vi "Untitled 3.vi"() -> ()   [LabVIEW 2017]
uses:
  <vilib>/Platform/TimedLoop/XDataNode/timing_clust.ctl
  <vilib>/Platform/TimedLoop/XDataNode/nitl_modes.ctl
  <vilib>/Platform/TimedLoop/XDataNode/wakeup.ctl
  <vilib>/myRIO/Common/Instrument Driver Framework/myRIO v1.0/UART/vis/myRIO v1.0 Close UART.vi
  Projects/Auto control/Global 1.vi
  Projects/Auto control/Outputs.vi
  Projects/Auto control/Inputs.vi
  <vilib>/myRIO/Common/Instrument Driver Framework/Utilities/vis/FPGA Ref Manager.vi
  <vilib>/myRIO/Common/Instrument Driver Framework/myRIO v1.0/myRIO v1.0 Reset FPGA.vi
  <vilib>/myRIO/Common/Instrument Driver Framework/myRIO v1.0/IRQ/vis/myRIO v1.0 IRQ Info FGV.vi
  <vilib>/myRIO/Common/Instrument Driver Framework/myRIO v1.0/IRQ/vis/myRIO v1.0 Timer IRQ Info FGV.vi
  <vilib>/myRIO/Common/Instrument Driver Framework/myRIO v1.0/IRQ/vis/myRIO v1.0 ISR Agent.vi
  <vilib>/platform/TimedLoop/XDataNode/XDataNode.xnode
  <vilib>/Platform/TimedLoop/XDataNode/XDNodeRunTimeDep.lvlib
  <vilib>/myRIO/Instrument Drivers/Utilities/Utilities.lvlib
panel:
  out "error out":errorcluster
  in  "Stop":bool
  out "Step":i16
  in  "Start":bool
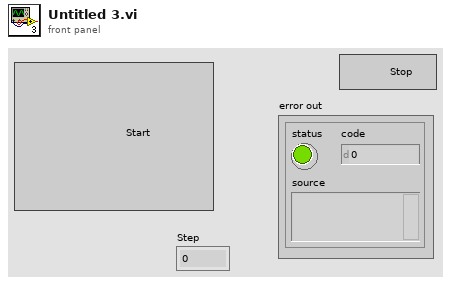
[diagram p1: front panel]
types:
  T1 = typedef "XDNodeRunTimeDep.lvlib/timing_clust.ctl" = cluster{"Expected End [f-1]":u64, "Actual End [f-1]":u64, "Finished Late? [f-1]":bool, "Expected End [i-1]":u64, "Actual End [i-1]":u64, "Finished Late? [i-1]":bool, "Expected Start [i]":u64, "Actual Start [i]":u64, "Expected Start [f]":u64, "Actual Start [f]":u64, "Source Name":string, "Structure Name":string, "Period":i64, "Deadline":i64, "Offset":i64, "Start":i64, "Priority":i32, "Timeout":i32, "Mode":T2, "Wakeup Reason":T3, "Error":errorcluster, "Source Type":string, "Secondary Source Type":string, "Global End Time":u64, "Global Start Time":u64, "Frame Duration":u64, "Iteration Duration":u64, "Assigned CPU":i32, "I/O Scan Engine Mode":u32}
  T2 = typedef "XDNodeRunTimeDep.lvlib/nitl_modes.ctl" = enum32{"No Change", "Process missed periods, maintain original phase", "Discard missed periods, maintain original phase", "Process missed periods, ignore original phase", "Discard missed periods, ignore original phase"}
  T3 = typedef "XDNodeRunTimeDep.lvlib/wakeup.ctl" = enum32{"Normal", "Aborted", "Asynchronous wakeup", "Timing source error", "Timed loop error", "Timeout"}
  T4 = typedef "I2C.lvlib/I2C Reference.ctl" = cluster{"myRIO Reference":T5, "I2C Channels Enum":T9, "I2C Configuration":T10}
  T5 = typedef "myRIO Generic Hardware Reference.ctl" = cluster{"myRIO Model":T6, "myRIO Hardware Reference":T7}
  T6 = typedef "Hardware Version Enum.ctl" = enum16{"Unknown", "myRIO-1900", "myRIO-1950", "roboRIO", "NI ELVIS RIO CM"}
  T7 = typedef "myRIO v1.0 Reference.ctl" = cluster{"Generic FPGA Reference":T8, "Allow multiple opens":bool}
  T8 = typedef "Generic FPGA Reference.ctl" = refnum<k20>
  T9 = typedef "I2C Channels Enum.ctl" = enum16{"Not Connected", "A/I2C", "B/I2C", "I2C/I2C"}
  T10 = typedef "I2C.lvlib/I2C Configuration.ctl" = cluster{"I2C Transfer Rate":T11}
  T11 = typedef "I2C.lvlib/I2C Transfer Rate.ctl" = enum16{"Standard mode (100 kbps)", "Fast mode (400 kbps)"}
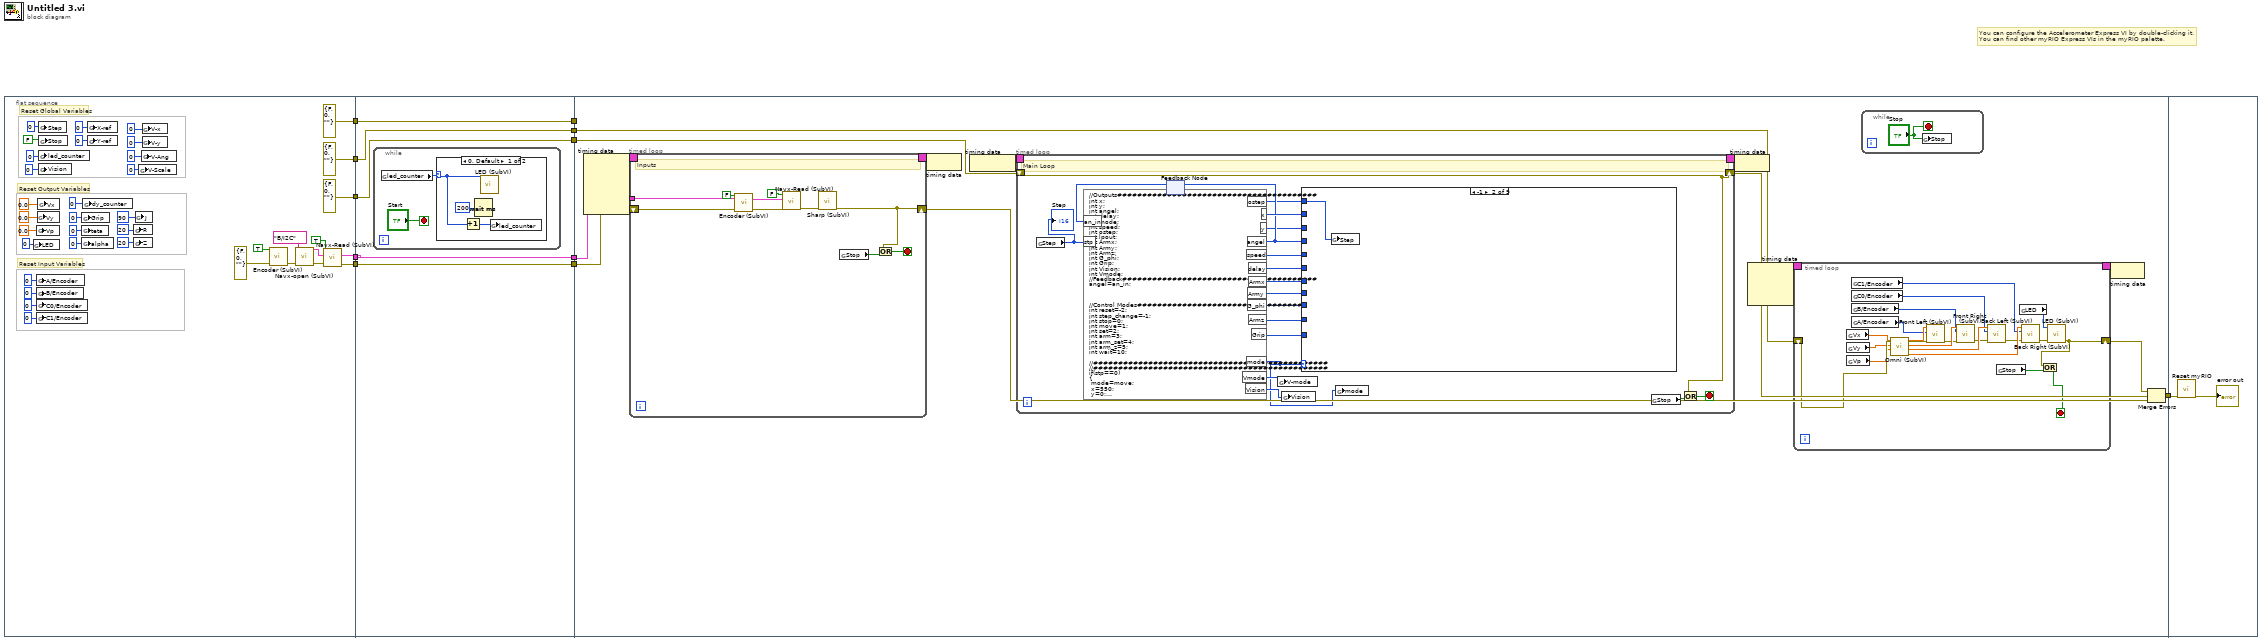
[diagram p0: block diagram]
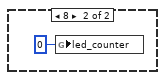
[diagram p2: hidden frame]
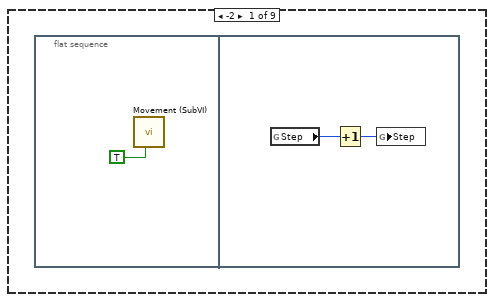
[diagram p3: hidden frame]
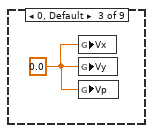
[diagram p4: hidden frame]
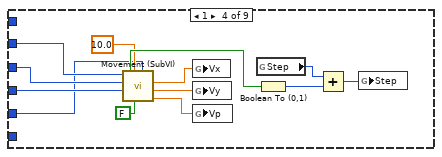
[diagram p5: hidden frame]
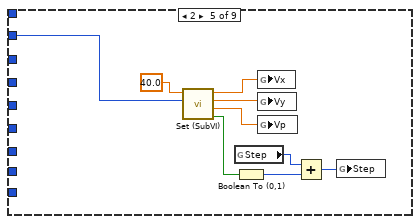
[diagram p6: hidden frame]
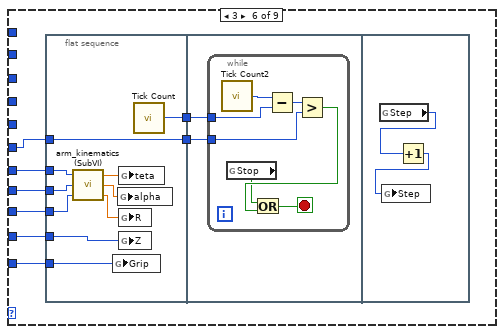
[diagram p7: hidden frame]
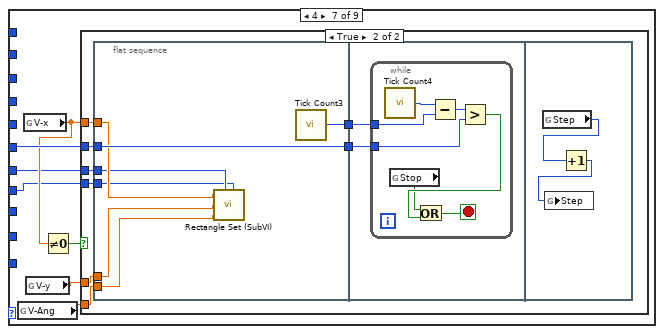
[diagram p8: hidden frame]
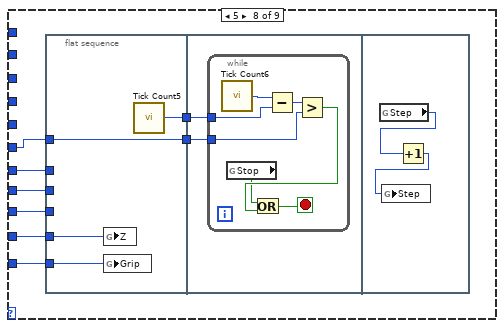
[diagram p10: hidden frame]
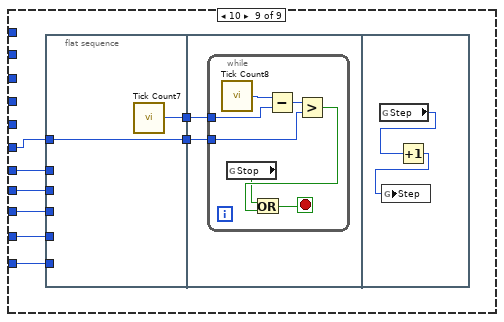
[diagram p11: hidden frame]
diagram:
  # "You can configure the Accelerometer Express VI by double-clicking it.\nYou can find other myRIO Express VIs in the myRIO palette."
  n1 = flat-sequence {
    tunnel: [w43] -> w11
    tunnel: [errorcluster {"status"=FALSE, "code"=0, "source"=""} ("error in (no error)")] -> w10
    tunnel: [errorcluster {"status"=FALSE, "code"=0, "source"=""} ("error in (no error)")] -> w9
    tunnel: [w41] -> w8
    tunnel: [errorcluster {"status"=FALSE, "code"=0, "source"=""} ("error in (no error)")] -> w7
    tunnel: w11 -> [w52]
    tunnel: [w52] -> w6
    tunnel: w10 -> [w51]
    tunnel: [w51] -> w5
    tunnel: w9 -> [w48]
    tunnel: w8 -> [w50]
    tunnel: [w50] -> w4
    tunnel: [w49] -> w3
    tunnel: w7 -> [w49]
    tunnel: [w48] -> w2
    tunnel: w6 -> [w72]
    tunnel: w5 -> [_]
    tunnel: w4 -> [w65]
    tunnel: w3 -> [w64]
    tunnel: [w63] -> w1
    tunnel: w2 -> [w59]
    tunnel: w1 -> [w267]
    frame #0 {
      # "Reset Global Variables"
      # "Reset Input Variables"
      # "Reset Output Variables"
      # "Initialize"
      n2 = global write "Outputs.vi" "LED"(i8 0 ("LED")) -> ()
      n3 = global write "Outputs.vi" "Vp"(0.0 ("Vp")) -> ()
      n4 = global write "Inputs.vi" "A/Encoder"(0 ("A/Encoder")) -> ()
      n5 = global write "Inputs.vi" "B/Encoder"(0 ("B/Encoder")) -> ()
      n6 = global write "Inputs.vi" "C0/Encoder"(0 ("C0/Encoder")) -> ()
      n7 = global write "Inputs.vi" "C1/Encoder"(0 ("C1/Encoder")) -> ()
      n8 = global write "Outputs.vi" "Vy"(0.0 ("Vy")) -> ()
      n9 = global write "Outputs.vi" "Vx"(0.0 ("Vx")) -> ()
      n10 = global write "Global 1.vi" "Step"(i16 0 ("Step")) -> ()
      n11 = global write "Global 1.vi" "led_counter"(i8 0 ("Step")) -> ()
      n12 = global write "Global 1.vi" "Vision"(i8 0 ("Step")) -> ()
      n13 = global write "Global 1.vi" "Stop"(FALSE ("Stop")) -> ()
      n14 = global write "Outputs.vi" "Grip"(i16 0 ("Grip")) -> ()
      n15 = global write "Outputs.vi" "teta"(i16 0 ("teta")) -> ()
      n16 = global write "Outputs.vi" "alpha"(i16 0 ("alpha")) -> ()
      n17 = global write "Outputs.vi" "dy_counter"(i8 0 ("LED")) -> ()
      n18 = global write "Global 1.vi" "X-ref"(i64 0 ("X-ref")) -> ()
      n19 = global write "Global 1.vi" "Y-ref"(i64 0 ("Y-ref")) -> ()
      n20 = global write "Outputs.vi" "R"(i16 20 ("R")) -> ()
      n21 = global write "Outputs.vi" "Z"(i16 20 ("Z")) -> ()
      n22 = global write "Outputs.vi" "J"(i16 90 ("J")) -> ()
      n23 = global write "Global 1.vi" "V-Scale"(i64 0 ("Y-ref")) -> ()
      n24 = global write "Global 1.vi" "V-Ang"(i64 0 ("X-ref")) -> ()
      n25 = global write "Global 1.vi" "V-x"(i64 0 ("X-ref")) -> ()
      n26 = global write "Global 1.vi" "V-y"(i64 0 ("Y-ref")) -> ()
      n27 = call "Encoder (SubVI).vi"("error in (no error)"=errorcluster {"status"=FALSE, "code"=0, "source"=""}, "Reset?"=TRUE ("Reset Counter")) -> ("error out"=w25:errorcluster)  [unwired: 9 in]
      n28 = call "Navx-open (SubVI).vi"("error in (no error)"=w25, "Channel Name"=tag "B/I2C") -> ("error out"=w45:errorcluster, "I2C Ref Out"=w41:T4)  [unwired: 8 in]
      n29 = call "Navx-Read (SubVI).vi"("error in (no error)"=w45, "I2C Ref Out"=w41, "Reset"=TRUE) -> ("error out"=w43:errorcluster)  [unwired: 7 in, 1 out]
    }
    frame #1 {
      n30 = while {
        stop <- "Start" stop-if-true
        n31 = global read "Global 1.vi" "led_counter"() -> (w53:i8)
        n32 = case shown="0, Default" w53 {
          selector: w53 -> [w55 _]
          frame 0, Default {
            n33 = Increment(x=w55) -> (x+1=w57:i8)
            n34 = Wait (ms)(milliseconds to wait=u32 200) -> ()  [unwired: 1 out]
            n35 = call "LED (SubVI).vi"("LED"=w55) -> ()  [unwired: 10 in, 1 out]
            n36 = global write "Global 1.vi" "led_counter"(w57) -> ()
          }
          frame 8 {
            n37 = global write "Global 1.vi" "led_counter"(i8 0 ("led_counter")) -> ()
          }
        }
      }
    }
    frame #2 {
      n38 = node-c288() -> (w67:T1)  [unwired: 5 in]
      n39 = timed-loop {
        shift-right: [w77] -> w62
        shift-left: w72 -> [w81]
        timing: w67 -> [_]
        timing-out: [_] -> w66
        tunnel: w65 -> [w79]
        stop <- w80 stop-if-true
        # "Inputs"
        n40 = call "Encoder (SubVI).vi"("error in (no error)"=w81, "Reset?"=FALSE ("Boolean")) -> ("error out"=w75:errorcluster)  [unwired: 9 in]
        n41 = call "Navx-Read (SubVI).vi"("error in (no error)"=w75, "I2C Ref Out"=w79, "Reset"=FALSE) -> ("error out"=w74:errorcluster)  [unwired: 7 in, 1 out]
        n42 = call "Sharp (SubVI).vi"("error in (no error)"=w74) -> ("error out"=w77:errorcluster)  [unwired: 10 in]
        n43 = global read "Global 1.vi" "Stop"() -> (w78:bool)
        n44 = Or(x=w77, y=w78) -> (x .or. y?=w80:bool)
      }
      n45 = node-c288(w66) -> ()
      n46 = node-c288() -> (w69:T1)
      n47 = timed-loop {
        shift-right: [w103] -> w61
        shift-left: w59 -> [w103]
        timing: w69 -> [_]
        timing-out: [_] -> w68
        stop <- w104 stop-if-true
        # "Main Loop"
        n48 = global read "Global 1.vi" "Step"() -> (w96:i16)
        "Step" <- w96
        n49 = feedback #1() -> (w100:i32)  [unwired: 1 in]
        n50 = formula code="//Outputs########################################\nint x;\nint y;\nint angel;\nint delay;\nint mode;\nint speed;\nint ostep;\nint lpout;\nint Armx;\nint Army;\nint Armz;\nint G_phi;\nint Grip;\nint Vision;\nint Vmode;\n//Feedback#######################################\nangel=an_in;\n\n\n\n//Control Modes##################################\nint reset=-2;\nint step_change=-1; \nint stop=0;\nint move=1;\nint set=2;\nint arm=3;\nint arm_set=4;\nint arm_z=5;\nint wait=10;\n\n//###############################################\n//###############################################\nif(stp==0)\n{\n\tmode=move;\n\tx=550;\n\ty=0;\n\tangel=0;\n\tspeed=100;\n}\nif(stp==1)\n{\n\tmode=move;\n\tx=0;\n\ty=-1400;\n\tangel=0;\n\tspeed=100;\n}\nif(stp==2)\n{\n\tmode=move;\n\tx=1400;\n\ty=0;\n\tangel=0;\n\tspeed=100;\n}\nif(stp==3)\n{\n\tmode=move;\n\tx=0;\n\ty=1400;\n\tangel=0;\n\tspeed=100;\n}\nif(stp==4)\n{\n\tmode=move;\n\tx=2000;\n\ty=0;\n\tangel=0;\n\tspeed=100;\n}\nif(stp==5)\n{\n\tmode=move;\n\tx=0;\n\ty=-1000;\n\tangel=0;\n\tspeed=100;\n}\nif(stp==6)\n{\n\tmode=move;\n\tx=2000;\n\ty=0;\n\tangel=0;\n\tspeed=100;\n}\nif(stp==7)\n{\n\tmode=move;\n\tx=0;\n\ty=0;\n\tangel=-90;\n\tspeed=100;\n}\nif(stp==8)\n{\n\tmode=move;\n\tx=4000;\n\ty=0;\n\tangel=0;\n\tspeed=100;\n}\n\n\nif(stp==9)\n{\n\tmode=stop;\n}"("stp"=w96, "an_in"=w100) -> ("x"=w102:i32, "y"=w97:i32, "mode"=w86:i32, "angel"=w99:i32, "delay"=w101:i32, "speed"=w98:i32, "ostep"=w94:i32, "Armx"=w92:i32, "Army"=w91:i32, "Armz"=w90:i32, "G_phi"=w93:i32, "Grip"=w89:i32, "Vision"=w88:i32, "Vmode"=w87:i32)
        n51 = feedback-in #1(w99) -> ()
        n52 = global write "Global 1.vi" "V-mode"(w87) -> ()
        n53 = global write "Global 1.vi" "Vision"(w88) -> ()
        n54 = case shown="-1" w86 {
          tunnel: w102 -> [_ _ _ w116 w131 _ _ _ _]
          tunnel: w97 -> [_ _ _ w115 _ _ _ _ _]
          tunnel: w99 -> [_ _ _ w114 _ _ _ _ _]
          tunnel: w101 -> [_ _ _ _ _ w138 w167 w200 w223]
          tunnel: w98 -> [_ _ _ w113 _ _ _ _ _]
          tunnel: w94 -> [_ w108 _ _ _ _ _ _ _]
          tunnel: w93 -> [_ _ _ _ _ w134 _ w196 w219]
          tunnel: w92 -> [_ _ _ _ _ w136 w162 w198 w221]
          tunnel: w91 -> [_ _ _ _ _ w135 w161 w197 w220]
          tunnel: w90 -> [_ _ _ _ _ w133 _ w195 w218]
          tunnel: w89 -> [_ _ _ _ _ w132 _ w194 w217]
          frame -2 {
            n55 = flat-sequence {
              frame #0 {
                n56 = call "Movement (SubVI).vi"("Reset"=TRUE) -> ()  [unwired: 6 in, 4 out]
              }
              frame #1 {
                n57 = global read "Global 1.vi" "Step"() -> (w107:i16)
                n58 = Increment(x=w107) -> (x+1=w106:i16)
                n59 = global write "Global 1.vi" "Step"(w106) -> ()
              }
            }
          }
          frame -1 {
            n60 = global write "Global 1.vi" "Step"(w108) -> ()
          }
          frame 0, Default {
            w109 = 0.0 ("Vy")
            n61 = global write "Outputs.vi" "Vx"(w109) -> ()
            n62 = global write "Outputs.vi" "Vy"(w109) -> ()
            n63 = global write "Outputs.vi" "Vp"(w109) -> ()
          }
          frame 1 {
            n64 = call "Movement (SubVI).vi"("Speed"=w113, "Reset"=FALSE, "Acc"=10.0, "Goal P"=w114, "Goal Y"=w115, "Goal X"=w116) -> ("Vp"=w118:dbl, "Vy"=w119:dbl, "Vx"=w120:dbl, "Reach?"=w121:bool)  [unwired: 1 in]
            n65 = global write "Outputs.vi" "Vx"(w120) -> ()
            n66 = global write "Outputs.vi" "Vy"(w119) -> ()
            n67 = global write "Outputs.vi" "Vp"(w118) -> ()
            n68 = global read "Global 1.vi" "Step"() -> (w110:i16)
            n69 = Boolean To (0,1)(Boolean=w121) -> (0, 1=w122:i16)
            n70 = Add(x=w110, y=w122) -> (x+y=w111:i16)
            n71 = global write "Global 1.vi" "Step"(w111) -> ()
          }
          frame 2 {
            n72 = call "Set (SubVI).vi"("Mode"=w131, "speed"=40.0) -> ("Reach?"=w123:bool, "Vp"=w127:dbl, "Vy"=w128:dbl, "Vx"=w129:dbl)  [unwired: 4 in]
            n73 = global read "Global 1.vi" "Step"() -> (w124:i16)
            n74 = Boolean To (0,1)(Boolean=w123) -> (0, 1=w126:i16)
            n75 = global write "Outputs.vi" "Vx"(w129) -> ()
            n76 = global write "Outputs.vi" "Vy"(w128) -> ()
            n77 = global write "Outputs.vi" "Vp"(w127) -> ()
            n78 = Add(x=w124, y=w126) -> (x+y=w125:i16)
            n79 = global write "Global 1.vi" "Step"(w125) -> ()
          }
          frame 3 {
            n80 = flat-sequence {
              tunnel: [w149] -> w139
              tunnel: w138 -> [w145]
              tunnel: [w145] -> w137
              tunnel: w136 -> [w144]
              tunnel: w135 -> [w143]
              tunnel: w134 -> [w142]
              tunnel: w133 -> [w141]
              tunnel: w132 -> [w140]
              tunnel: w139 -> [w151]
              tunnel: w137 -> [w150]
              frame #0 {
                n81 = call "arm_kinematics (SubVI).vi"("alpha"=w142, "y"=w143, "x"=w144) -> ("R"=w146:dbl, "alpha"=w147:dbl, "teta"=w148:dbl)
                n82 = global write "Outputs.vi" "Grip"(w140) -> ()
                n83 = global write "Outputs.vi" "alpha"(w147) -> ()
                n84 = global write "Outputs.vi" "teta"(w148) -> ()
                n85 = global write "Outputs.vi" "R"(w146) -> ()
                n86 = global write "Outputs.vi" "Z"(w141) -> ()
                n87 = call "Tick Count"() -> ("Tick Count(mSec)"=w149:u32)
              }
              frame #1 {
                n88 = while {
                  tunnel: w151 -> [w157]
                  tunnel: w150 -> [w152]
                  stop <- w154 stop-if-true
                  n89 = call "Tick Count2"() -> ("Tick Count(mSec)"=w158:u32)
                  n90 = global read "Global 1.vi" "Stop"() -> (w153:bool)
                  n91 = Subtract(x=w158, y=w157) -> (x-y=w156:u32)
                  n92 = Greater?(x=w156, y=w152) -> (0:w155:bool)
                  n93 = Or(x=w153, y=w155) -> (x .or. y?=w154:bool)
                }
              }
              frame #2 {
                n94 = global read "Global 1.vi" "Step"() -> (w159:i16)
                n95 = Increment(x=w159) -> (x+1=w160:i16)
                n96 = global write "Global 1.vi" "Step"(w160) -> ()
              }
            }
          }
          frame 4 {
            n97 = global read "Global 1.vi" "V-Ang"() -> (w163:sgl)
            n98 = global read "Global 1.vi" "V-x"() -> (w164:sgl)
            n99 = global read "Global 1.vi" "V-y"() -> (w166:sgl)
            n100 = Not Equal To 0?(x=w164) -> (x != 0?=w165:bool)
            n101 = case shown="True" w165 {
              tunnel: w167 -> [_ w173]
              tunnel: w166 -> [_ w172]
              tunnel: w164 -> [_ w171]
              tunnel: w163 -> [_ w170]
              tunnel: w162 -> [_ w169]
              tunnel: w161 -> [_ w168]
              frame False {
              }
              frame True {
                n102 = flat-sequence {
                  tunnel: [w182] -> w175
                  tunnel: w173 -> [w181]
                  tunnel: [w181] -> w174
                  tunnel: w172 -> [w179]
                  tunnel: w171 -> [w180]
                  tunnel: w170 -> [w178]
                  tunnel: w169 -> [w177]
                  tunnel: w168 -> [w176]
                  tunnel: w175 -> [w184]
                  tunnel: w174 -> [w183]
                  frame #0 {
                    n103 = call "Rectangle Set (SubVI).vi"("x"=w180, "x in"=w177, "y"=w179, "alpha"=w178, "y in"=w176) -> ()  [unwired: 6 in]
                    n104 = call "Tick Count3"() -> ("Tick Count(mSec)"=w182:u32)
                  }
                  frame #1 {
                    n105 = while {
                      tunnel: w184 -> [w190]
                      tunnel: w183 -> [w185]
                      stop <- w187 stop-if-true
                      n106 = call "Tick Count4"() -> ("Tick Count(mSec)"=w191:u32)
                      n107 = global read "Global 1.vi" "Stop"() -> (w186:bool)
                      n108 = Subtract(x=w191, y=w190) -> (x-y=w189:u32)
                      n109 = Greater?(x=w189, y=w185) -> (0:w188:bool)
                      n110 = Or(x=w186, y=w188) -> (x .or. y?=w187:bool)
                    }
                  }
                  frame #2 {
                    n111 = global read "Global 1.vi" "Step"() -> (w192:i16)
                    n112 = Increment(x=w192) -> (x+1=w193:i16)
                    n113 = global write "Global 1.vi" "Step"(w193) -> ()
                  }
                }
              }
            }
          }
          frame 5 {
            n114 = flat-sequence {
              tunnel: [w205] -> w201
              tunnel: w200 -> [w204]
              tunnel: [w204] -> w199
              tunnel: w198 -> [_]
              tunnel: w197 -> [_]
              tunnel: w196 -> [_]
              tunnel: w195 -> [w203]
              tunnel: w194 -> [w202]
              tunnel: w201 -> [w207]
              tunnel: w199 -> [w206]
              frame #0 {
                n115 = global write "Outputs.vi" "Z"(w203) -> ()
                n116 = global write "Outputs.vi" "Grip"(w202) -> ()
                n117 = call "Tick Count5"() -> ("Tick Count(mSec)"=w205:u32)
              }
              frame #1 {
                n118 = while {
                  tunnel: w207 -> [w213]
                  tunnel: w206 -> [w208]
                  stop <- w210 stop-if-true
                  n119 = call "Tick Count6"() -> ("Tick Count(mSec)"=w214:u32)
                  n120 = global read "Global 1.vi" "Stop"() -> (w209:bool)
                  n121 = Subtract(x=w214, y=w213) -> (x-y=w212:u32)
                  n122 = Greater?(x=w212, y=w208) -> (0:w211:bool)
                  n123 = Or(x=w209, y=w211) -> (x .or. y?=w210:bool)
                }
              }
              frame #2 {
                n124 = global read "Global 1.vi" "Step"() -> (w215:i16)
                n125 = Increment(x=w215) -> (x+1=w216:i16)
                n126 = global write "Global 1.vi" "Step"(w216) -> ()
              }
            }
          }
          frame 10 {
            n127 = flat-sequence {
              tunnel: [w226] -> w224
              tunnel: w223 -> [w225]
              tunnel: [w225] -> w222
              tunnel: w221 -> [_]
              tunnel: w220 -> [_]
              tunnel: w219 -> [_]
              tunnel: w218 -> [_]
              tunnel: w217 -> [_]
              tunnel: w224 -> [w228]
              tunnel: w222 -> [w227]
              frame #0 {
                n128 = call "Tick Count7"() -> ("Tick Count(mSec)"=w226:u32)
              }
              frame #1 {
                n129 = while {
                  tunnel: w228 -> [w234]
                  tunnel: w227 -> [w229]
                  stop <- w231 stop-if-true
                  n130 = call "Tick Count8"() -> ("Tick Count(mSec)"=w235:u32)
                  n131 = global read "Global 1.vi" "Stop"() -> (w230:bool)
                  n132 = Subtract(x=w235, y=w234) -> (x-y=w233:u32)
                  n133 = Greater?(x=w233, y=w229) -> (0:w232:bool)
                  n134 = Or(x=w230, y=w232) -> (x .or. y?=w231:bool)
                }
              }
              frame #2 {
                n135 = global read "Global 1.vi" "Step"() -> (w236:i16)
                n136 = Increment(x=w236) -> (x+1=w237:i16)
                n137 = global write "Global 1.vi" "Step"(w237) -> ()
              }
            }
          }
        }
        n138 = global write "Global 1.vi" "mode"(w86) -> ()
        n139 = global read "Global 1.vi" "Stop"() -> (w95:bool)
        n140 = Or(x=w103, y=w95) -> (x .or. y?=w104:bool)
      }
      n141 = node-c288(w68) -> ()
      n142 = node-c288() -> (w71:T1)  [unwired: 3 in]
      n143 = timed-loop {
        timing: w71 -> [_]
        timing-out: [_] -> w70
        shift-right: [w259] -> w60
        shift-left: w64 -> [w260]
        stop <- w261 stop-if-true
        n144 = global read "Outputs.vi" "Vx"() -> (w255:dbl)
        n145 = global read "Outputs.vi" "Vy"() -> (w257:dbl)
        n146 = global read "Outputs.vi" "Vp"() -> (w256:dbl)
        n147 = global read "Inputs.vi" "C1/Encoder"() -> (w248:i32)
        n148 = global read "Inputs.vi" "C0/Encoder"() -> (w247:i32)
        n149 = global read "Inputs.vi" "B/Encoder"() -> (w246:i32)
        n150 = global read "Inputs.vi" "A/Encoder"() -> (w245:i32)
        n151 = call "Omni (SubVI).vi"("Vp"=w256, "Vy"=w257, "Vx"=w255) -> ("Back_Right"=w253:dbl, "Back_Left"=w258:dbl, "Front_Right"=w254:dbl, "Front_Left"=w251:dbl)  [unwired: 4 in]
        n152 = call "Front Left (SubVI).vi"("setpoint"=w251, "Counter Value"=w245, "error in"=w260) -> ("error out"=w252:errorcluster)  [unwired: 6 in, 1 out]
        n153 = call "Front Right (SubVI).vi"("error in"=w252, "Counter Value"=w246, "setpoint"=w254) -> ("error out"=w250:errorcluster)  [unwired: 7 in, 1 out]
        n154 = call "Back Left (SubVI).vi"("error in"=w250, "Counter Value"=w247, "setpoint"=w258) -> ("error out"=w249:errorcluster)  [unwired: 7 in, 1 out]
        n155 = global read "Global 1.vi" "Stop"() -> (w244:bool)
        n156 = global read "Outputs.vi" "LED"() -> (w242:i8)
        n157 = call "Back Right (SubVI).vi"("error in"=w249, "Counter Value"=w248, "setpoint"=w253) -> ("error out"=w243:errorcluster)  [unwired: 7 in, 1 out]
        n158 = call "LED (SubVI).vi"("error in (no error)"=w243, "LED"=w242) -> ("error out"=w259:errorcluster)  [unwired: 9 in]
        n159 = Or(x=w259, y=w244) -> (x .or. y?=w261:bool)
      }
      n160 = while {
        stop <- "Stop" stop-if-true
        n161 = global write "Global 1.vi" "Stop"("Stop") -> ()
      }
      n162 = node-c288(w70) -> ()
      n163 = Merge Errors(w60, w61, w62) -> (w63:errorcluster)
    }
    frame #3 {
      # "Close"
      n164 = call <vilib>:"Reset myRIO.vi"("error in (no error)"=w267) -> ("error out"=→"error out":errorcluster)  [unwired: 10 in]
    }
  }
